vi "IsLinkedToLibraryorClass.vi"(8 "error in (no error)":errorcluster, 10 "CheckChangedLibrariesOnly":bool=TRUE, 11 "Workspace Path":path=path "C:/sw-deps-monitor") -> (0 "error out":errorcluster, 3 "Status Indicator":string)   [LabVIEW 2019, in "DepsWatch.lvlib"]
uses:
  DepsWatch.lvlib
  28450a76-a9d3-48c7-9439-369bd691228e.vi
  <vilib>/JDP Science/JSONtext/Variant to JSON Text.vi
  <vilib>/Wiresmith Technology/G CLI/CLI Class/CLI.lvclass
  <vilib>/JDP Science/JSONtext/LVClass Serializer/JSONtext LVClass Serializer.lvclass
  <vilib>/SLL Toolkit/SLL String/SLL String.lvlib
  <vilib>/JDP Science/JSONtext/JSONtext.lvlib
panel:
  in  "GUI Mode? {F)":bool
  in  "Tab Control":enum32{"GUI Mode", "CLI Mode"}(tab)
  out "Args":string[](array[string])=["C:\\sw-deps-monitor", "True"]
  # "When in GUI Mode, the controls will be used, \nIn CLI Mode, the Args will be used"
  # "Workspace Path"
  # "CheckChangedLibrariesOnly? True/False"
  # "Command to run the VI from terminal\ng-cli -v --lv-ver 2023 --arch 32 \"C:\\sw-deps-monitor\\CICD\\AutomatedChecks\\IsLinkedToLibrary.vi\" -- \"C:\\sw-deps-monitor\" \"False\""
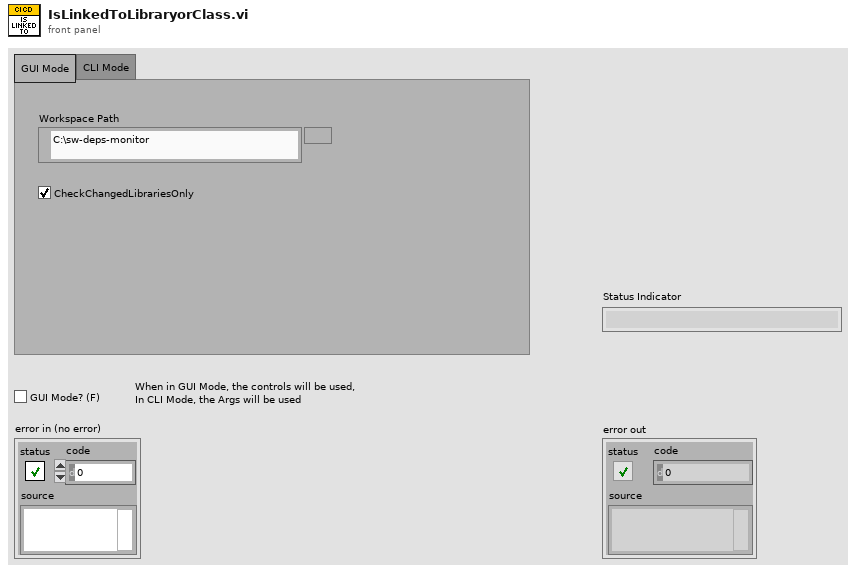
[diagram p1: front panel]
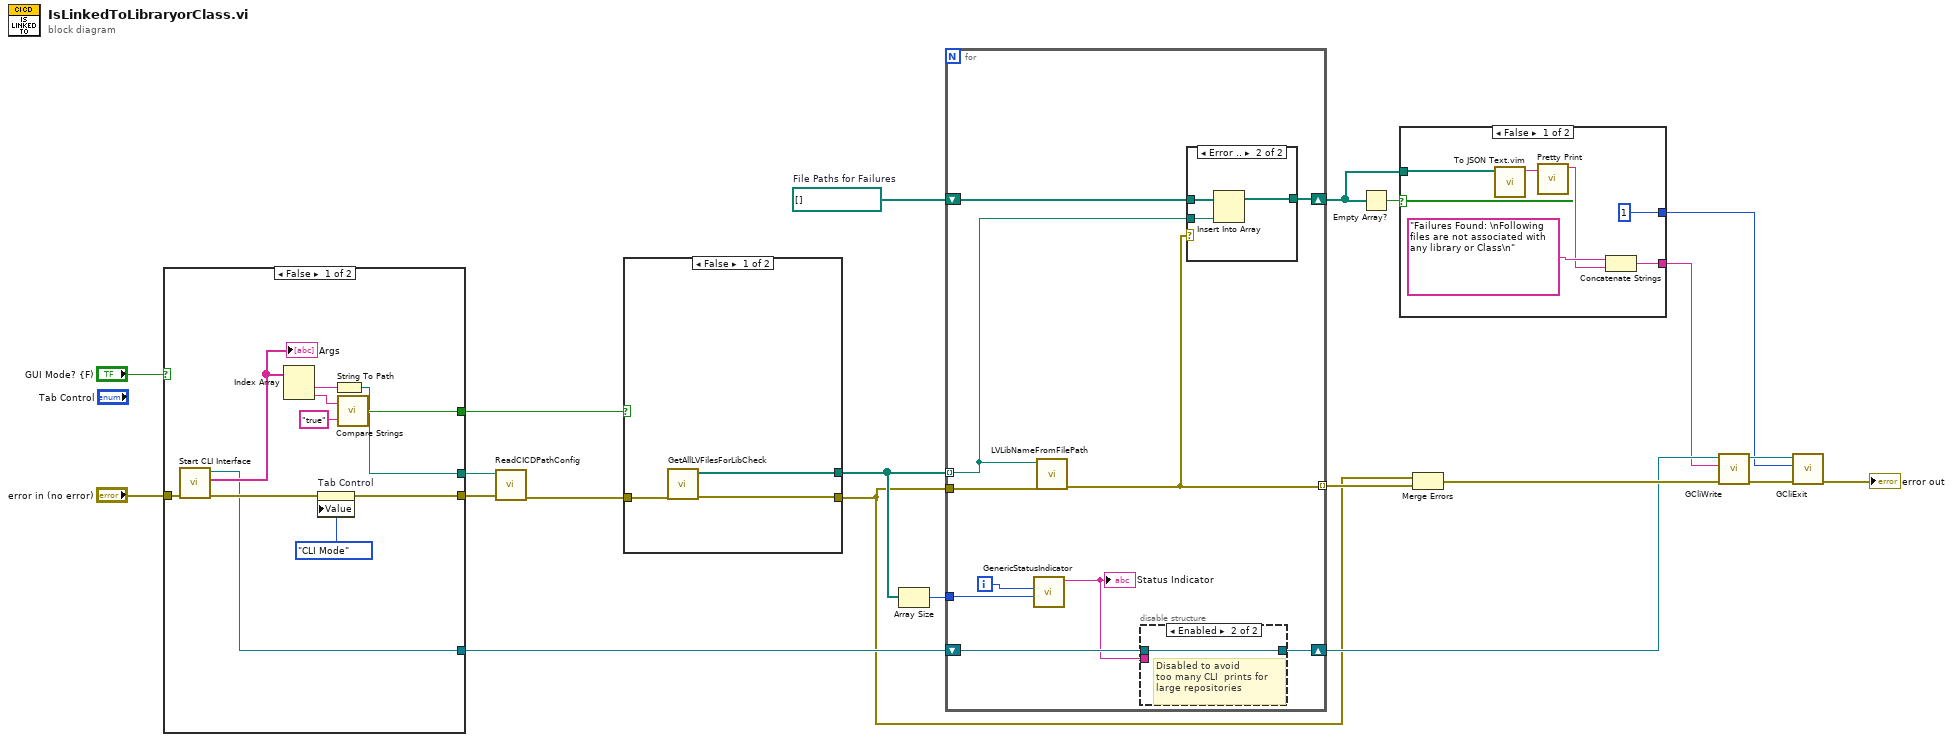
[diagram p0: block diagram]
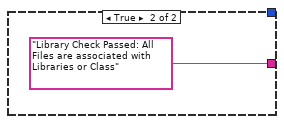
[diagram p2: hidden frame]
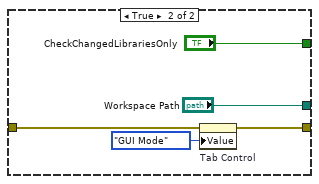
[diagram p3: hidden frame]
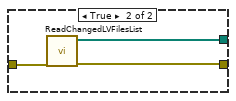
[diagram p4: hidden frame]
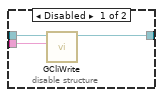
[diagram p5: hidden frame]
diagram:
  w2 = path[] []  # File Paths for Failures
  n1 = case shown="False" "GUI Mode? {F)" {
    tunnel: "error in (no error)" -> [w32 w35]
    tunnel: [w29 w34] -> w13
    tunnel: [w25 "CheckChangedLibrariesOnly"] -> w14
    tunnel: [w24 "Workspace Path"] -> w12
    tunnel: [w22 _] -> w11
    frame False {
      n2 = call <vilib>:"Start CLI Interface.vi"("error in (no error)"=w32) -> ("error out"=w31:errorcluster, "Custom Parameters"=w23:string[], "CLI out"=w22:refnum<class "CLI.lvclass">)  [unwired: 7 in, 1 out]
      "Args" <- w23
      n3 = Index Array(array=w23) -> (element #1=w28:string, element #2=w27:string)  [unwired: 2 in]
      n4 = property on="Tab Control" class="TabCtl (strict)"(error in=w31, "Value"=enum32{"GUI Mode", "CLI Mode"}."CLI Mode" ("Tab Control")) -> (error out=w29:errorcluster)  [unwired: 1 in, 1 out]
      n5 = String To Path(string=w28) -> (path=w24:path)
      n6 = call <vilib>:"Compare Strings.vi"("y"="true", "x"=w27) -> ("Equal?"=w25:bool)
    }
    frame True {
      n7 = property on="Tab Control" class="TabCtl (strict)"(error in=w35, "Value"=enum32{"GUI Mode", "CLI Mode"}."GUI Mode" ("Tab Control")) -> (error out=w34:errorcluster)  [unwired: 1 in, 1 out]
    }
  }
  n8 = call "ReadCICDPathConfig.vi"("error in (no error)"=w13, "Workspace Path"=w12) -> ("error out"=w17:errorcluster)  [unwired: 8 in, 1 out]
  n9 = case shown="False" w14 {
    tunnel: w17 -> [w40 w43]
    tunnel: [w38 w41] -> w19
    tunnel: [w39 w42] -> w1
    frame False {
      n10 = call "GetAllLVFilesForLibCheck.vi"("error in (no error)"=w40) -> ("error out"=w39:errorcluster, "LV File paths (VIs, CTLs, LVCLASSes)"=w38:path[])  [unwired: 9 in]
    }
    frame True {
      n11 = call "ReadChangedLVFilesList.vi"("error in (no error)"=w43) -> ("error out"=w42:errorcluster, "ChangedLVFilesList"=w41:path[])  [unwired: 9 in]
    }
  }
  n12 = Array Size(array=w19) -> (size(s)=w18:i32)
  n13 = for {
    tunnel: w1 -> [w48]
    tunnel: w19 -> [w44] mode=indexing
    tunnel: [w47] -> w21 mode=indexing
    tunnel: w18 -> [w53]
    shift-right: [w45] -> w6
    shift-left: w2 -> [w46]
    shift-right: [w50] -> w9
    shift-left: w11 -> [w51]
    i -> [w52]
    n14 = call "GenericStatusIndicator.vi"("Total"=w53, "Current Iteration"=w52) -> ("CLI Status to Print"=w49:string)  [unwired: 9 in]
    "Status Indicator" <- w49
    n15 = call "LVLibNameFromFilePath.vi"("error in (no error)"=w48, "LV File Path"=w44) -> ("error out"=w47:errorcluster)  [unwired: 8 in, 1 out]
    n16 = disable-structure shown="Enabled" {
      disable-tunnel: w51 -> [w56 w57]
      disable-tunnel: [w55 w57] -> w50
      disable-tunnel: w49 -> [w54 _]
      frame Disabled {
        n17 = call "GCliWrite.vi"("Text to Write"=w54, "CLI in"=w56) -> ("CLI out"=w55:refnum<class "CLI.lvclass">)  [unwired: 8 in, 1 out]
      }
      frame Enabled {
        # "Disabled to avoid\ntoo many CLI  prints for \nlarge repositories"
      }
    }
    n18 = case shown="Error .." w47 {
      tunnel: w46 -> [w58 w61]
      tunnel: w44 -> [_ w60]
      tunnel: [w58 w59] -> w45
      frame No Error {
      }
      frame Error {
        n19 = Insert Into Array(array=w61, new element=w60) -> (w59:path[])  [unwired: 1 in]
      }
    }
  }
  n20 = Empty Array?(array=w6) -> (empty?=w7:bool)
  n21 = case shown="False" w7 {
    tunnel: w6 -> [w66 _]
    tunnel: [w65 "Library Check Passed: All Files are associated with Libraries or Class"] -> w5
    tunnel: [1 _] -> w3
    frame False {
      n22 = call "To JSON Text.vim"("Anything"=w66) -> ("<JSON>"=w63:string)  [unwired: 9 in, 1 out]
      n23 = call <vilib>:"Pretty Print.vi"("JSON"=w63) -> ("<JSON>"=w62:string)  [unwired: 8 in, 2 out]
      n24 = Concatenate Strings("Failures Found: \nFollowing files are not associated with any library or Class\n" ("string"), w62) -> (w65:string)
    }
    frame True {
    }
  }
  n25 = Merge Errors(w1, w21) -> (w20:errorcluster)
  n26 = call "GCliWrite.vi"("error in (no error)"=w20, "Text to Write"=w5, "CLI in"=w9) -> ("error out"=w10:errorcluster, "CLI out"=w8:refnum<class "CLI.lvclass">)  [unwired: 7 in]
  n27 = call "GCliExit.vi"("error in (no error)"=w10, "No Error Code (0)"=w3, "CLI in"=w8) -> ("error out"=→"error out":errorcluster)  [unwired: 8 in]
